vi "SweepConfig.vi"(8 "error in (no error)":errorcluster, 9 "Sweep Time (s)":dbl, 10 "Num Points":u32, 11 "SpecA_MXA in":refnum<class "SpecA_MXA.lvclass">) -> (0 "error out":errorcluster, 3 "SpecA_MXA out":refnum<class "SpecA_MXA.lvclass">)   [LabVIEW 2014, in "SpecA_MXA.lvclass"]
uses:
  SpecA_MXA.lvclass
  SpecA_MXA.lvclass/SpecA_MXA.ctl
  <instrlib>/Agilent MXA Series/Agilent MXA Series.lvlib
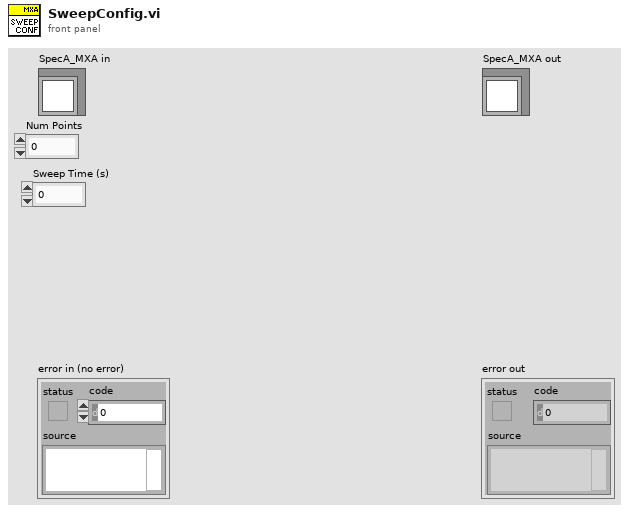
[diagram p1: front panel]
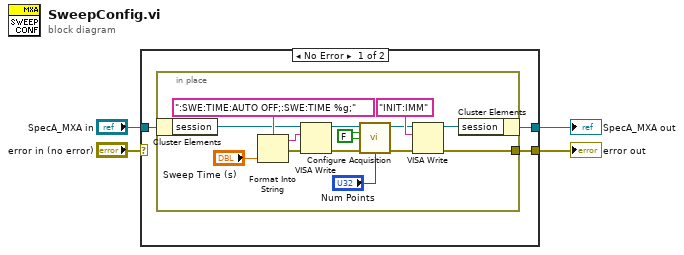
[diagram p0: block diagram]
diagram:
  n1 = case shown="No Error" "error in (no error)" {
    selector: "error in (no error)" -> [_ w23]
    tunnel: [w7 w23] -> w4
    tunnel: "SpecA_MXA in" -> [w6 w22]
    tunnel: [w5 w22] -> w2
    frame No Error {
      n2 = in-place {
        in-place-border: [w14] -> w7
        w20 = FALSE ("Enable Continuous Sweep (T: Enable)")
        n3 = in-place-cluster #1(w6) -> ("session"=w8:refnum<visa-resource-name>)
        n4 = Format Into String(format string=":SWE:TIME:AUTO OFF;:SWE:TIME %g;" ("write buffer"), "Sweep Time (s)") -> (resulting string=w21:string, error out=w13:errorcluster)  [unwired: 2 in]
        n5 = VISA Write(VISA resource name=w8, write buffer=w21, error in (no error)=w13) -> (VISA resource name out=w19:refnum<visa-resource-name>, error out=w12:errorcluster)  [unwired: 1 out]
        n6 = call <instrlib>:"Configure Acquisition.vi"("VISA resource name"=w19, "Enable Continuous Sweep (T: Enable)"=w20, "Auto Detector (T: Enable)"=w20, "error in (no error)"=w12, "Sweep Points (1001)"="Num Points") -> ("VISA resource name out"=w16:refnum<visa-resource-name>, "error out"=w17:errorcluster)  [unwired: 9 in]
        n7 = VISA Write(VISA resource name=w16, write buffer="INIT:IMM" ("format string"), error in (no error)=w17) -> (VISA resource name out=w11:refnum<visa-resource-name>, error out=w14:errorcluster)  [unwired: 1 out]
        n8 = in-place-cluster #1("session"=w11) -> (w5:refnum<class "SpecA_MXA.lvclass">)
      }
    }
    frame Error {
    }
  }
  "error out" <- w4
  "SpecA_MXA out" <- w2
